vi "Trust Incorrect Server Identity.vi"(8 "error in (no error)":errorcluster, 11 "client in":refnum<class "Generic Client.lvclass">) -> (0 "error out":errorcluster, 2 "permanent?":bool, 3 "client out":refnum<class "Generic Client.lvclass">)   [LabVIEW 2020, in "NI_SSH.lvlib" / "Generic Client.lvclass"]
doc: "USE OF THIS FUNCTION MAY CAUSE YOUR SYSTEMS TO BECOME COMPROMISED.\nDO NOT USE THIS FUNCTION WITHOUT THE EXPRESS AND INFORMED CONSENT OF THE USER. \nNATIONAL INSTRUMENTS IS NOT LIABLE FOR DAMAGES CAUSED BY MISUSE OF THIS FUNCTION.\n\nExplicitly trust the identity of a server, even if it does not match the previously known server identity.\n\nThis can only be called after an SFTP connection attempt has failed. Otherwise, this VI will return an error."
uses:
  <vilib>/net/SSH/Client/Generic/Generic Client.lvclass
  <vilib>/Utility/error.llb/Error Cluster From Error Code.vi
  <vilib>/ErrorRing/Error Ring.xnode
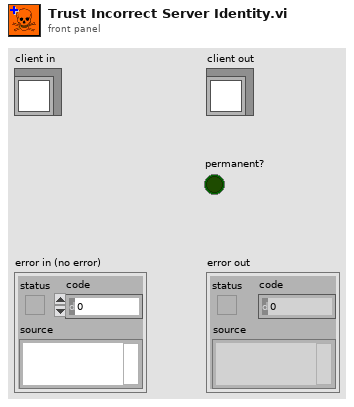
[diagram p1: front panel]
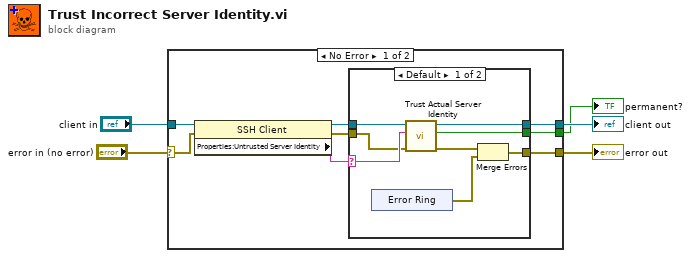
[diagram p0: block diagram]
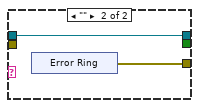
[diagram p2: hidden frame]
diagram:
  n1 = case shown="No Error" "error in (no error)" {
    selector: "error in (no error)" -> [w8 w33]
    tunnel: [w12 w33] -> w2
    tunnel: "client in" -> [w10 w32]
    tunnel: [w13 w32] -> w3
    tunnel: [w6 _] -> w1
    frame No Error {
      n2 = property class="SSH Client"(reference=w10, error in=w8) -> (reference out=w11:refnum<class "Generic Client.lvclass">, error out=w7:errorcluster, "Properties:Untrusted Server Identity"=w9:string)
      n3 = case shown="Default" w9 {
        selector: w9 -> [w20 _]
        tunnel: w11 -> [w21 w27]
        tunnel: [w19 w27] -> w13
        tunnel: w7 -> [w18 _]
        tunnel: [w15 w26] -> w12
        tunnel: [w14 _] -> w6
        frame Default {
          n4 = xnode "Error Ring"() -> ("error out"=w16:errorcluster)
          n5 = call-dynamic "Trust Actual Server Identity.vi"("error in (no error)"=w18, "fingerprint"=w20, "SSH Client in"=w21) -> ("error out"=w17:errorcluster, "permanent?"=w14:bool, "SSH Client out"=w19:refnum<class "Generic Client.lvclass">)  [unwired: 6 in]
          n6 = Merge Errors(w17, w16) -> (w15:errorcluster)
        }
        frame "" {
          n7 = xnode "Error Ring"() -> ("error out"=w26:errorcluster)
        }
      }
    }
    frame Error {
    }
  }
  "error out" <- w2
  "client out" <- w3
  "permanent?" <- w1
